vi "Resolve Zip Destination.vi"(8 "error in (no error)":errorcluster, 11 "Zip File In":path) -> (0 "error out":errorcluster, 2 "Destination":path, 3 "Zip File Out":path)   [LabVIEW 2019, in "Archivist.lvclass"]
uses:
  Archivist.lvclass
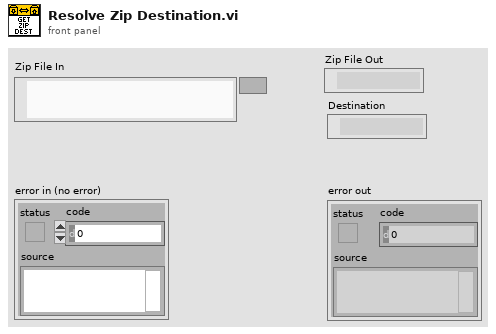
[diagram p1: front panel]
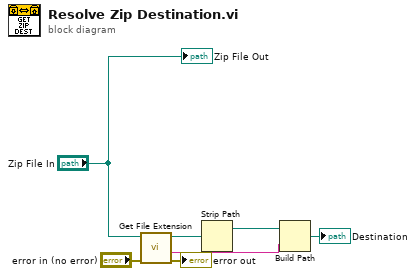
[diagram p0: block diagram]
diagram:
  n1 = call <vilib>:"Get File Extension.vi"("error in (no error)"="error in (no error)", "file"="Zip File In") -> ("error out"=→"error out":errorcluster, "filename without extension"=w5:string, "dup file"=w7:path)  [unwired: 5 in, 2 out]
  n2 = Strip Path(path=w7) -> (stripped path=w6:path)  [unwired: 1 out]
  n3 = Build Path(base path=w6, name or relative path=w5) -> (appended path=→"Destination":path)
  "Zip File Out" <- "Zip File In"
